vi "isDiscoverAliveBye.vi"(1 "input":string) -> (0 "output":string)   [LabVIEW 2010]
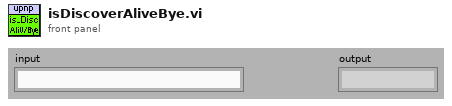
[diagram p1: front panel]
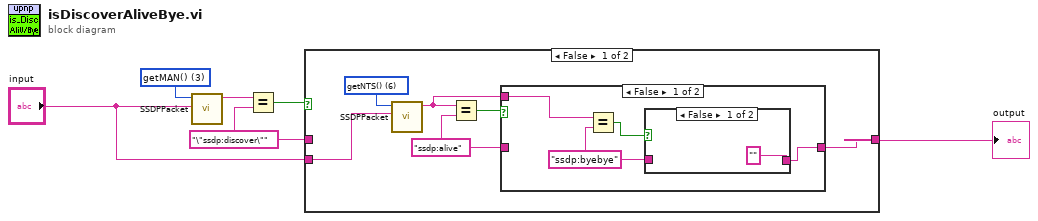
[diagram p0: block diagram]
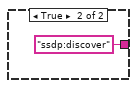
[diagram p4: hidden frame]
diagram:
  w3 = "\"ssdp:discover\""
  w6 = u16 3 items=["getHost()", "getCacheControl()", "getLocation()", "getMAN()", "getST()", "getNT()", "getNTS()", "getServer()", "getUSN()", "getMX()"] ("getMethods")
  n1 = call "SSDPPacket.vi"("data"="input", "getMethods"=w6) -> ("value"=w5:string)  [unwired: 9 out]
  n2 = Equal?(x=w5, y=w3) -> (x = y?=w4:bool)
  n3 = case shown="False" w4 {
    tunnel: w3 -> [_ _]
    tunnel: [w8 "ssdp:discover"] -> w2
    tunnel: "input" -> [w11 _]
    frame False {
      w9 = "ssdp:alive"
      w12 = u16 6 items=["getHost()", "getCacheControl()", "getLocation()", "getMAN()", "getST()", "getNT()", "getNTS()", "getServer()", "getUSN()", "getMX()"] ("getMethods")
      n4 = call "SSDPPacket.vi"("data"=w11, "getMethods"=w12) -> ("value"=w7:string)  [unwired: 9 out]
      n5 = Equal?(x=w7, y=w9) -> (x = y?=w10:bool)
      n6 = case shown="False" w10 {
        tunnel: w9 -> [_ w19]
        tunnel: [w13 w19] -> w8
        tunnel: w7 -> [w16 _]
        frame False {
          w14 = "ssdp:byebye"
          n7 = Equal?(x=w16, y=w14) -> (x = y?=w15:bool)
          n8 = case shown="False" w15 {
            tunnel: w14 -> [_ w18]
            tunnel: ["" w18] -> w13
            frame False {
            }
            frame True {
            }
          }
        }
        frame True {
        }
      }
    }
    frame True {
    }
  }
  "output" <- w2
